vi "Copy Value.vi"(10 "From":refnum<class "Type.lvclass">, 11 "Integer in":refnum<class "Integer.lvclass">) -> (2 "error out":errorcluster, 3 "Integer out":refnum<class "Integer.lvclass">)   [LabVIEW 2020, in "Conditum.lvlib" / "Columns.lvlib" / "Integer.lvclass"]
uses:
  Integer.lvclass
  C:/dev/lv20CE/lv-conditum/Conditum/Columns/Type/Type.lvclass
  Type/Type.lvclass
  Integer.lvclass/Integer.ctl
  Type/Type.lvclass/Type.ctl
  Type/Clear NULL.vi
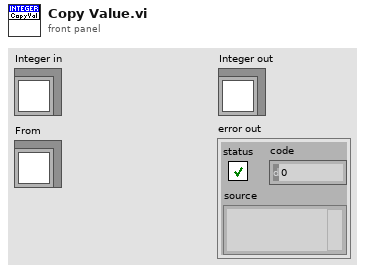
[diagram p1: front panel]
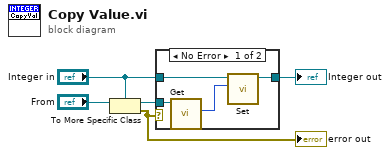
[diagram p0: block diagram]
diagram:
  n1 = To More Specific Class(target class="Integer in", reference="From") -> (specific class reference=w5:refnum<class "Integer.lvclass">, error out=w1:errorcluster)  [unwired: 1 in]
  "error out" <- w1
  n2 = case shown="No Error" w1 {
    tunnel: w5 -> [w9 _]
    tunnel: "Integer in" -> [w7 w10]
    tunnel: [w6 w10] -> w4
    frame No Error {
      n3 = call "Get.vi"("Integer in"=w9) -> ("Value"=w8:i64)  [unwired: 10 in]
      n4 = call "Set.vi"("Value"=w8, "Integer in"=w7) -> ("Integer out"=w6:refnum<class "Integer.lvclass">)  [unwired: 9 in]
    }
    frame Error {
    }
  }
  "Integer out" <- w4
